vi "Update_DestDir_For_Main_Dest_Change.vi"(8 "error in (no error)":errorcluster, 11 "AB_DepDLL in":refnum<class "AB_DepDLL.lvclass">) -> (0 "error out":errorcluster, 3 "AB_DepDLL out":refnum<class "AB_DepDLL.lvclass">)   [LabVIEW 2020, in "AB_DepDLL.lvclass"]
uses:
  <vilib>/AppBuilder/AB_Classes/DepDLL/AB_DepDLL.lvclass
  e:/builds/penguin/labview/branches/2020/dev/dist/vi.lib/AppBuilder/AB_Classes/Build/AB_Build.lvclass
  <vilib>/AppBuilder/AB_Classes/Deployment/AB_Deployment.lvlib
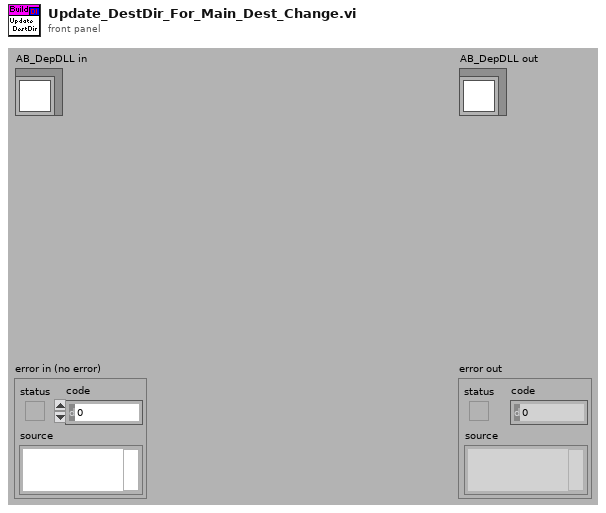
[diagram p1: front panel]
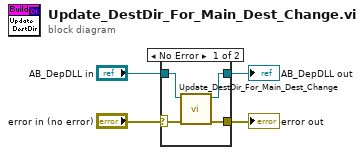
[diagram p0: block diagram]
diagram:
  n1 = case shown="No Error" "error in (no error)" {
    selector: "error in (no error)" -> [w6 w10]
    tunnel: [w5 w10] -> w1
    tunnel: [w7 w9] -> w4
    tunnel: "AB_DepDLL in" -> [w8 w9]
    frame No Error {
      n2 = call <vilib>:"Update_DestDir_For_Main_Dest_Change.vi"("error in (no error)"=w6, "Build in"=w8) -> ("error out"=w5:errorcluster, "Build out"=w7:refnum<class "AB_DepDLL.lvclass">)  [unwired: 8 in]
    }
    frame Error {
    }
  }
  "error out" <- w1
  "AB_DepDLL out" <- w4
